vi "HENON.VI"(4 "IV:y":dbl format="%.8f", 5 "IV: x":dbl format="%.8f", 6 "B":dbl=0.30000000000000004 format="%.8f", 7 "A":dbl=1.4 format="%.8f", 8 "Number of Iterates to compute":dbl=10000.0, 9 "Number of pre-iterates":dbl=300.0 format="%.2f") -> (0 "Y.s":dbl[](array[numeric]) format="%.2f", 1 "X's":dbl[](array[numeric]) format="%.2f", 2 "FinalY":dbl=-0.1670038898051678 format="%.8f", 3 "Final X":dbl=0.8905758143832117 format="%.8f")   [LabVIEW 2012]
panel:
  out "?":cluster{dbl[], dbl[]}(graph)
  # "2"
  # "{"
  # "Xn+1 = Yn +1-AXn"
  # "The Henon Map:"
  # "Yn+1 = BXn"
  # "VI Inputs"
  # "Yn vs Xn"
  # "Outputs"
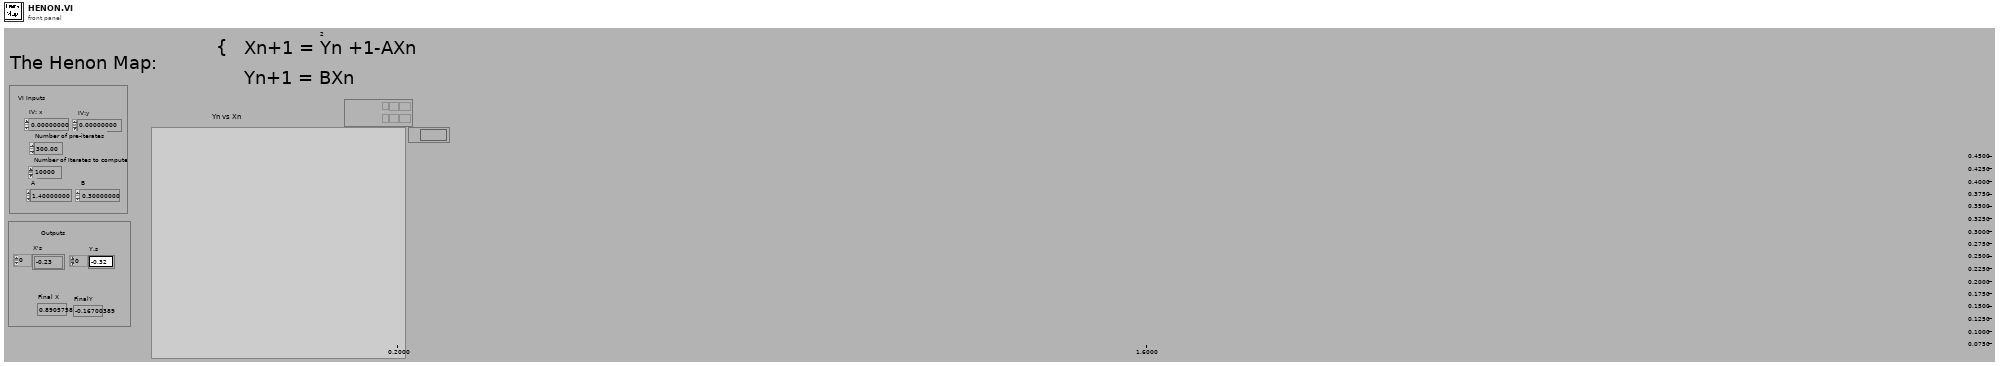
[diagram p1: front panel]
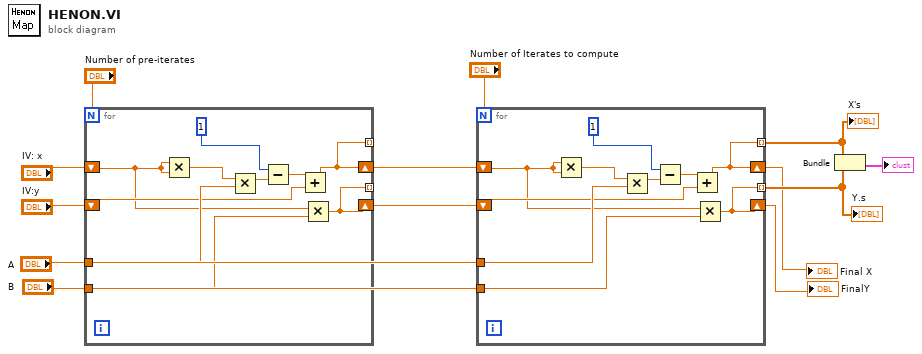
[diagram p0: block diagram]
diagram:
  n1 = for {
    N: "Number of pre-iterates" -> [_]
    shift-right: [w15] -> w7
    shift-left: "IV: x" -> [w16]
    tunnel: "A" -> [w22]
    tunnel: "B" -> [w18]
    shift-right: [w14] -> w6
    shift-left: "IV:y" -> [w17]
    tunnel: [w15] -> _ mode=indexing
    tunnel: [w14] -> _ mode=indexing
    n2 = Multiply(x=w16, y=w16) -> (x*y=w21:dbl)
    n3 = Multiply(x=w21, y=w22) -> (x*y=w20:dbl)
    n4 = Subtract(x=1, y=w20) -> (x-y=w19:dbl)
    n5 = Add(x=w19, y=w17) -> (x+y=w15:dbl)
    n6 = Multiply(x=w16, y=w18) -> (x*y=w14:dbl)
  }
  n7 = for {
    N: "Number of Iterates to compute" -> [_]
    shift-right: [w25] -> w1
    shift-left: w7 -> [w26]
    tunnel: "A" -> [w32]
    tunnel: "B" -> [w28]
    shift-right: [w24] -> w2
    shift-left: w6 -> [w27]
    tunnel: [w25] -> w11 mode=indexing
    tunnel: [w24] -> w10 mode=indexing
    n8 = Multiply(x=w26, y=w26) -> (x*y=w31:dbl)
    n9 = Multiply(x=w31, y=w32) -> (x*y=w30:dbl)
    n10 = Subtract(x=1, y=w30) -> (x-y=w29:dbl)
    n11 = Add(x=w29, y=w27) -> (x+y=w25:dbl)
    n12 = Multiply(x=w26, y=w28) -> (x*y=w24:dbl)
  }
  "Final X" <- w1
  "FinalY" <- w2
  "X's" <- w11
  "Y.s" <- w10
  n13 = Bundle(w11, w10) -> (→"?":cluster{dbl[], dbl[]})  [unwired: 1 in]
